vi "Write In Chain.vi"(10 "Add to":T1, 11 "Interlock in":refnum<class "Interlock.lvclass">) -> (3 "Interlock out":refnum<class "Interlock.lvclass">)   [LabVIEW 2015, in "Interlocks.lvlib" / "Interlock.lvclass"]
uses:
  Interlock.lvclass
  Controls/Add IL to -Enumerator.ctl
  Interlock.lvclass/Interlock.ctl
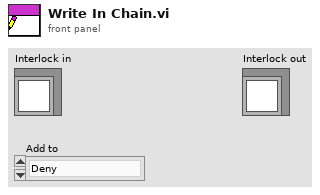
[diagram p1: front panel]
types:
  T1 = typedef "Add IL to -Enumerator.ctl" = enum16{"Deny", "Allow", "None"}
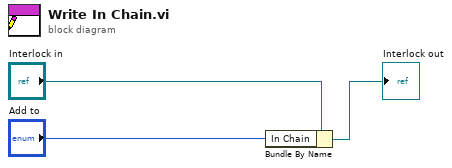
[diagram p0: block diagram]
diagram:
  n1 = Bundle By Name(cluster="Interlock in", "In Chain"="Add to") -> (→"Interlock out":refnum<class "Interlock.lvclass">)
